vi "ExecuteCommand.vi"() -> ()   [LabVIEW 2017]
uses:
  <resource>/objmgr/DOMUserDefRef.rc
panel:
  in  "Node":string
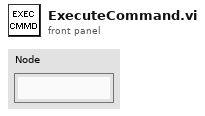
[diagram p1: front panel]
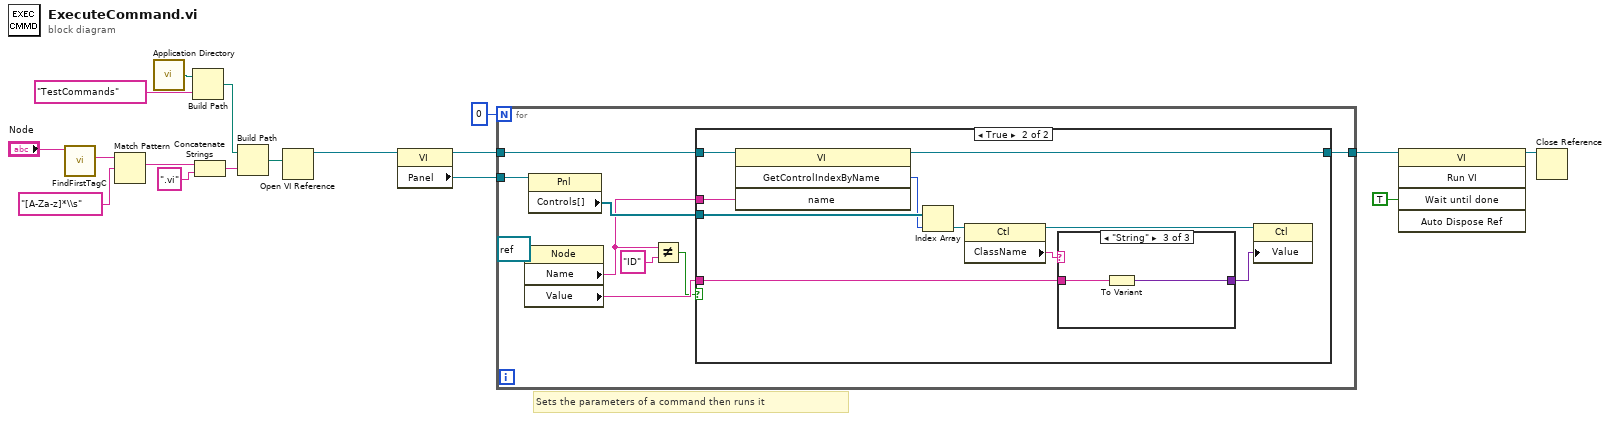
[diagram p0: block diagram]
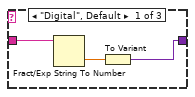
[diagram p3: hidden frame]
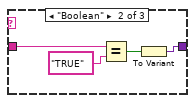
[diagram p4: hidden frame]
diagram:
  # "Sets the parameters of a command then runs it"
  n1 = call "FindFirstTagC.vi"("XML String In"="Node") -> ("tag"=w5:string)  [unwired: 1 in, 9 out]
  n2 = Match Pattern(string=w5, regular expression="[A-Za-z]*\\s") -> (match substring=w2:string)  [unwired: 1 in, 3 out]
  n3 = call <vilib>:"Application Directory.vi"() -> ("Application Directory"=w17:path)
  n4 = Build Path(base path=w17, name or relative path="TestCommands") -> (appended path=w15:path)
  n5 = Concatenate Strings(w2, ".vi" ("string")) -> (w13:string)
  n6 = Build Path(base path=w15, name or relative path=w13) -> (appended path=w12:path)
  n7 = Open VI Reference(vi path=w12) -> (vi reference=w11:refnum<vi>)  [unwired: 5 in, 1 out]
  n8 = property class="VI"(reference=w11) -> (reference out=w9:refnum<vi>, "Panel"=w7:refnum<vi>)  [unwired: 1 in, 1 out]
  n9 = for {
    N: 0 -> [_]
    tunnel: w9 -> [w25]
    tunnel: [w26] -> w8
    tunnel: w7 -> [w24]
    n10 = property class="Node"(reference=refnum<k20> refnum ("Node")) -> ("Name"=w21:string, "Value"=w22:string)  [unwired: 1 in, 2 out]
    n11 = property class="Pnl"(reference=w24) -> ("Controls[]"=w23:refnum<vi>[])  [unwired: 1 in, 2 out]
    n12 = Not Equal?(x=w21, y="ID") -> (x != y?=w19:bool)
    n13 = case shown="True" w19 {
      tunnel: [w27 w37] -> w26
      tunnel: w25 -> [w27 w36]
      tunnel: w23 -> [_ w35]
      tunnel: w22 -> [_ w31]
      tunnel: w21 -> [_ w28]
      frame False {
      }
      frame True {
        n14 = invoke class="VI" method="GetControlIndexByName"(reference=w36, "name"=w28) -> (reference out=w37:refnum<vi>, "GetControlIndexByName"=w34:i32)  [unwired: 2 in, 2 out]
        n15 = Index Array(array=w35, index=w34) -> (element=w33:refnum<vi>)
        n16 = property class="Ctl"(reference=w33) -> (reference out=w30:refnum<vi>, "ClassName"=w32:string)  [unwired: 1 in, 1 out]
        n17 = case shown="\"String\"" w32 {
          tunnel: [w39 w42 w46] -> w29
          tunnel: w31 -> [w38 w41 w45]
          frame "Digital", Default {
            n18 = Fract/Exp String To Number(string=w38) -> (number=w40:dbl)  [unwired: 3 in, 1 out]
            n19 = To Variant(anything=w40) -> (Variant=w39:variant)
          }
          frame "Boolean" {
            n20 = Equal?(x=w41, y="TRUE") -> (x = y?=w43:bool)
            n21 = To Variant(anything=w43) -> (Variant=w42:variant)
          }
          frame "String" {
            n22 = To Variant(anything=w45) -> (Variant=w46:variant)
          }
        }
        n23 = property class="Ctl"(reference=w30, "Value"=w29) -> ()  [unwired: 1 in, 2 out]
      }
    }
  }
  n24 = invoke class="VI" method="Run VI"(reference=w8, "Wait until done"=TRUE ("Wait Until Done")) -> (reference out=w6:refnum<vi>)  [unwired: 3 in, 4 out]
  n25 = Close Reference(reference=w6) -> ()  [unwired: 1 in, 1 out]
